vi "Actor Core.vi"(8 "error in":errorcluster, 11 "SlideView In":refnum<class "SlideView.lvclass">) -> (0 "error out":errorcluster, 3 "Actor out":refnum<class "Actor.lvclass">)   [LabVIEW 2017, in "MVA Example.lvlib" / "SlideView.lvclass"]
doc: "(<B>Filename</B>: Actor Framework.lvlib:Actor.lvclass:Actor Core.vi)\n\nReceives messages to the actor, reacts to them, and initiates any error handling that may shut the actor down.\n\nDescendant classes may override this VI to append parallel tasks for the actor to complete while it handles messages. Overrides use the Call Parent Method node.\n\n<License>\nCopyright © 2017 Composed Systems, LLC | All rights reserved\nwww.composed.io\n\nAuthor: Ethan Stern <ethan.stern@composed.io>\n\nThis software is provided \"AS IS\" WITHOUT WARRANTIES, either express or implied, AND IS FOR EDUCATIONAL PURPOSES ONLY.\n</License>MVA Framework 1.6.0.31\nEthan Stern - Composed Systems\nCopyright (c) 2018, Composed Systems"
uses:
  SlideView.lvclass
  <vilib>/ActorFramework/Actor/Actor.lvclass
  <vilib>/Composed Systems/MVA Framework/Framework/IViewable/IViewable/IViewable.lvclass
panel:
  out "Vertical Slider 2":dbl(slide) caption="Vertical Slider" scale=0.0..10.0 scale format="%#2_2g"
  out "Vertical Slider":dbl(slide) scale=0.0..10.0 scale format="%#2_2g"
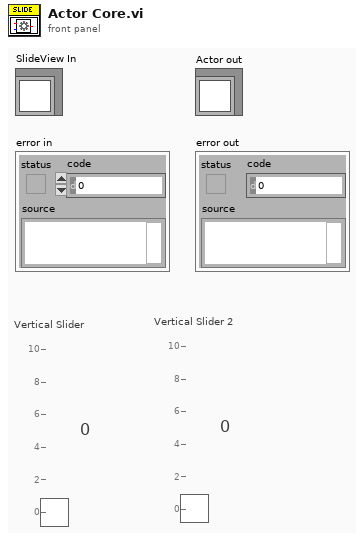
[diagram p1: front panel]
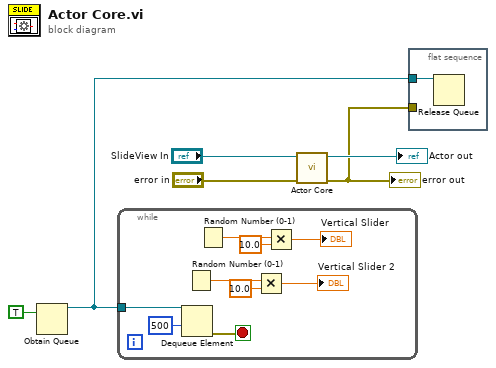
[diagram p0: block diagram]
diagram:
  n1 = Obtain Queue(element data type=TRUE) -> (queue out=w2:refnum<queue>)  [unwired: 4 in, 2 out]
  n2 = while {
    tunnel: w2 -> [w15]
    stop <- w13 stop-if-true
    n3 = Dequeue Element(queue=w15, timeout in ms (-1)=500) -> (error out=w13:errorcluster)  [unwired: 1 in, 3 out]
    n4 = Random Number (0-1)() -> (number: 0 to 1=w12:dbl)
    n5 = Random Number (0-1)() -> (number: 0 to 1=w9:dbl)
    n6 = Multiply(x=w12, y=10.0) -> (x*y=→"Vertical Slider 2":dbl)
    n7 = Multiply(x=w9, y=10.0) -> (x*y=→"Vertical Slider":dbl)
  }
  n8 = call-parent "Actor Core.vi"("error in"="error in", "IViewable In"="SlideView In") -> ("error out"=w1:errorcluster, "Actor out"=→"Actor out":refnum<class "Actor.lvclass">)  [unwired: 8 in]
  "error out" <- w1
  n9 = flat-sequence {
    tunnel: w2 -> [w16]
    tunnel: w1 -> [_]
    frame #0 {
      n10 = Release Queue(queue=w16) -> ()  [unwired: 2 in, 3 out]
    }
  }
